vi "fgv_NtripClient_stop.vi"(7 "cmd":T1, 11 "local stops":T2) -> (3 "local stops out":T2)   [LabVIEW 2019]
uses:
  Ctrl/cmd_ini-RW.ctl
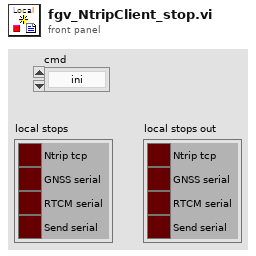
[diagram p1: front panel]
types:
  T1 = typedef "cmd_ini-RW.ctl" = enum16{"ini", "read", "write"}
  T2 = cluster{"Ntrip tcp":bool, "GNSS serial":bool, "RTCM serial":bool, "Send serial":bool}
  T3 = cluster{"Ntrip tcp":bool, "GNSS serial":bool, "RTCM serial":bool, "Extra serial":bool}
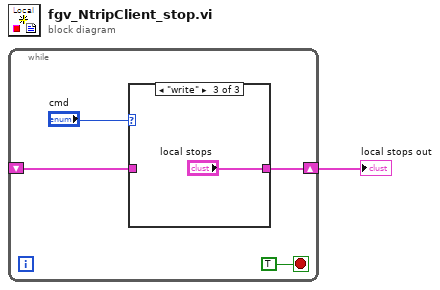
[diagram p0: block diagram]
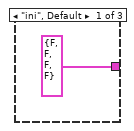
[diagram p2: hidden frame]
diagram:
  n1 = while {
    shift-right: [w4] -> w1
    shift-left: _ -> [w3]
    stop <- TRUE stop-if-true
    n2 = case shown="\"write\"" "cmd" {
      tunnel: [T3 {"Ntrip tcp"=FALSE, "GNSS serial"=FALSE, "RTCM serial"=FALSE, "Extra serial"=FALSE} ("local stops") w7 "local stops"] -> w4
      tunnel: w3 -> [_ w7 _]
      frame "ini", Default {
      }
      frame "read" {
      }
      frame "write" {
      }
    }
  }
  "local stops out" <- w1
